vi "Adjust_Image_Quality.vi"() -> ()   [LabVIEW 2017]
uses:
  <vilib>/userdefined/High Color/IMAQdx.ctl
  <resource>/objmgr/imaqdx.rc
panel:
  out "Within Range":bool
  out "Image":T1(plugin-control)
  out "error out":errorcluster
  in  "Session In":T2
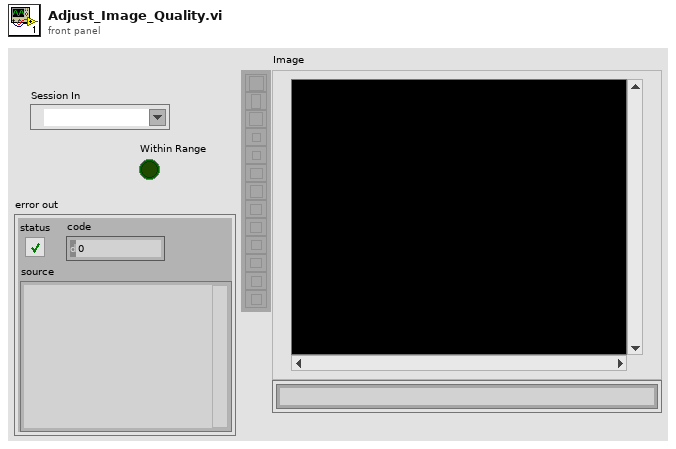
[diagram p1: front panel]
types:
  T1 = typedef "IMAQ Image.ctl" = refnum<image>
  T2 = typedef "IMAQdx.ctl" = refnum<k21>
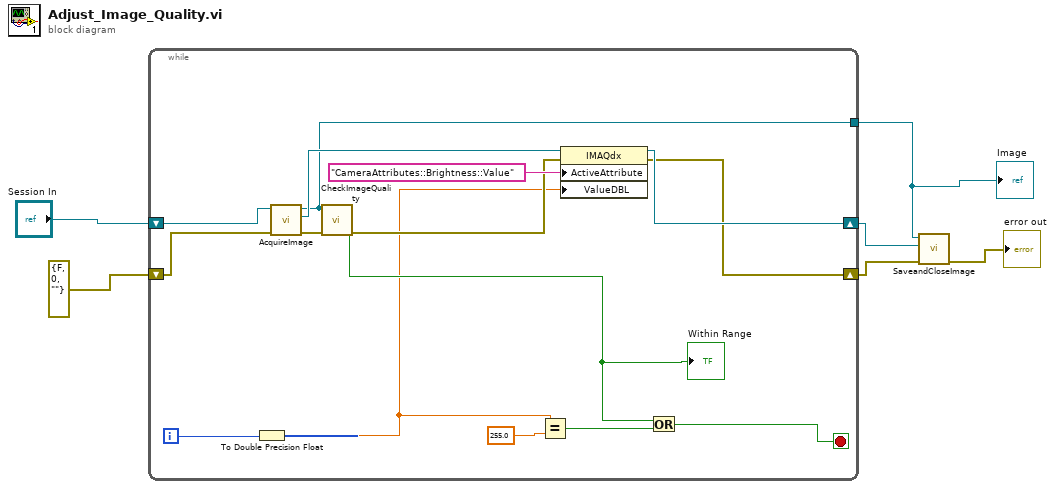
[diagram p0: block diagram]
diagram:
  n1 = while {
    shift-right: [w10] -> w3
    shift-left: "Session In" -> [w15]
    shift-right: [w9] -> w4
    shift-left: errorcluster {"status"=FALSE, "code"=0, "source"=""} ("error out") -> [w7]
    tunnel: [w12] -> w2
    i -> [w18]
    stop <- w20 stop-if-true
    n2 = To Double Precision Float(number=w18) -> (double precision float=w8:dbl)
    n3 = call "AcquireImage.vi"("error in"=w7, "Session In"=w15) -> ("error out"=w16:errorcluster, "Session Out"=w13:T2, "Image"=w12:T1)  [unwired: 7 in]
    n4 = call "CheckImageQuality.vi"("error in (no error)"=w16, "Image"=w12) -> ("error out"=w14:errorcluster, "Within Range"=w11:bool)  [unwired: 5 in, 3 out]
    "Within Range" <- w11
    n5 = Equal?(x=w8, y=255.0) -> (x = y?=w17:bool)
    n6 = property class="IMAQdx"(reference=w13, error in=w14, "ActiveAttribute"="CameraAttributes::Brightness::Value", "ValueDBL"=w8) -> (reference out=w10:T2, error out=w9:errorcluster)
    n7 = Or(x=w11, y=w17) -> (x .or. y?=w20:bool)
  }
  "Image" <- w2
  n8 = call "SaveandCloseImage.vi"("error in"=w4, "Session In"=w3, "Image In"=w2) -> ("error out"=→"error out":errorcluster)  [unwired: 8 in]
